vi "niDTS WLAN INSTR RX Close.vi"(8 "error in (no error)":errorcluster, 11 "niDTS WLAN INSTR RX in":refnum<class "niDTS WLAN INSTR RX.lvclass">) -> (0 "error out":errorcluster)   [LabVIEW 2015, in "niDTS WLAN.lvlib" / "niDTS WLAN INSTR RX.lvclass"]
uses:
  niDTS WLAN INSTR RX.lvclass
  niDTS WLAN INSTR RX.lvclass/niDTS WLAN INSTR RX.ctl
  RiviInstDriver/InstDriver/Objects/InstDriver.lvclass
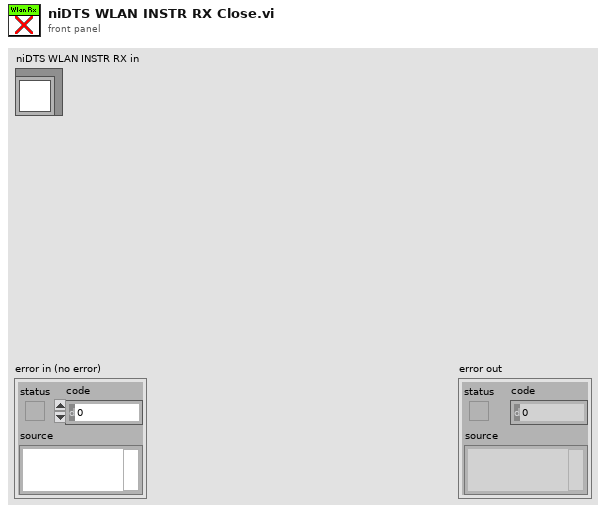
[diagram p1: front panel]
types:
  T1 = typedef "niRfsgWlan.lvclass/niRfsgWlan INC Handle.ctl" = refnum<data-value>
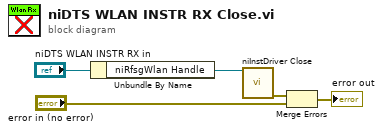
[diagram p0: block diagram]
diagram:
  n1 = Unbundle By Name("niDTS WLAN INSTR RX in") -> ("niRfsgWlan Handle"=w2:T1)
  n2 = call "niInstDriver Close.vi"("InstDriver Handle in"=w2) -> ("error out"=w1:errorcluster)  [unwired: 14 in]
  n3 = Merge Errors(w1, "error in (no error)") -> (→"error out":errorcluster)
